vi "LS DAS File Save.vi"(0 "Raw Data":fxp<+/-,22,11>[](array[numeric]), 1 "ValidFifoRead":bool, 2 "Day In":i32, 3 "Count In":i32, 4 "Bank1 Filepath":path, 5 "Bank2 Filepath":path, 6 "Opens In":i32[](array[numeric]), 7 "Row Count In":i32, 8 "Bank2Slow":bool, 9 "LowRate":i32, 10 "Anomaly Filepath":path) -> (15 "Day Out":i32, 18 "Count Out":i32, 19 "Second File Count Out":i32)   [LabVIEW 2013]
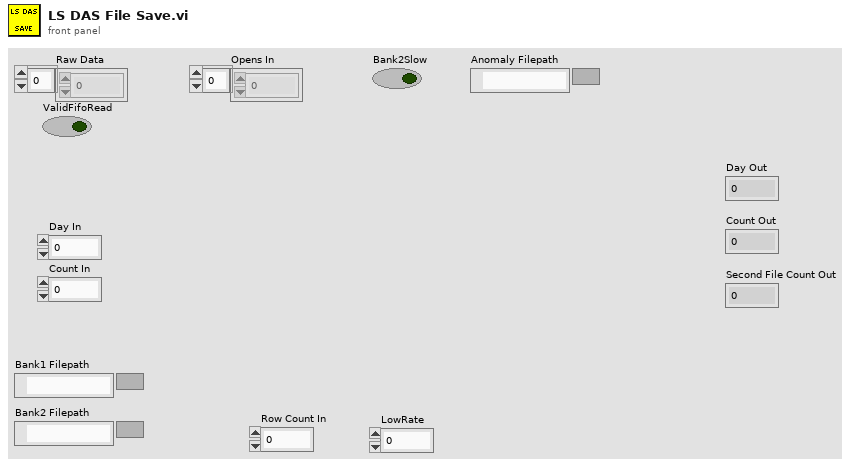
[diagram p1: front panel]
types:
  T1 = enum16{"open", "replace", "create", "open or create", "replace or create", "replace or create with confirmation"}
  T2 = typedef "LVDateTimeRec.ctl" = cluster{"fractional second":dbl, "second":i32, "minute":i32, "hour":i32, "day of month":i32, "month":i32, "year":i32, "day of week":i32, "day of year":i32, "DST":i32}
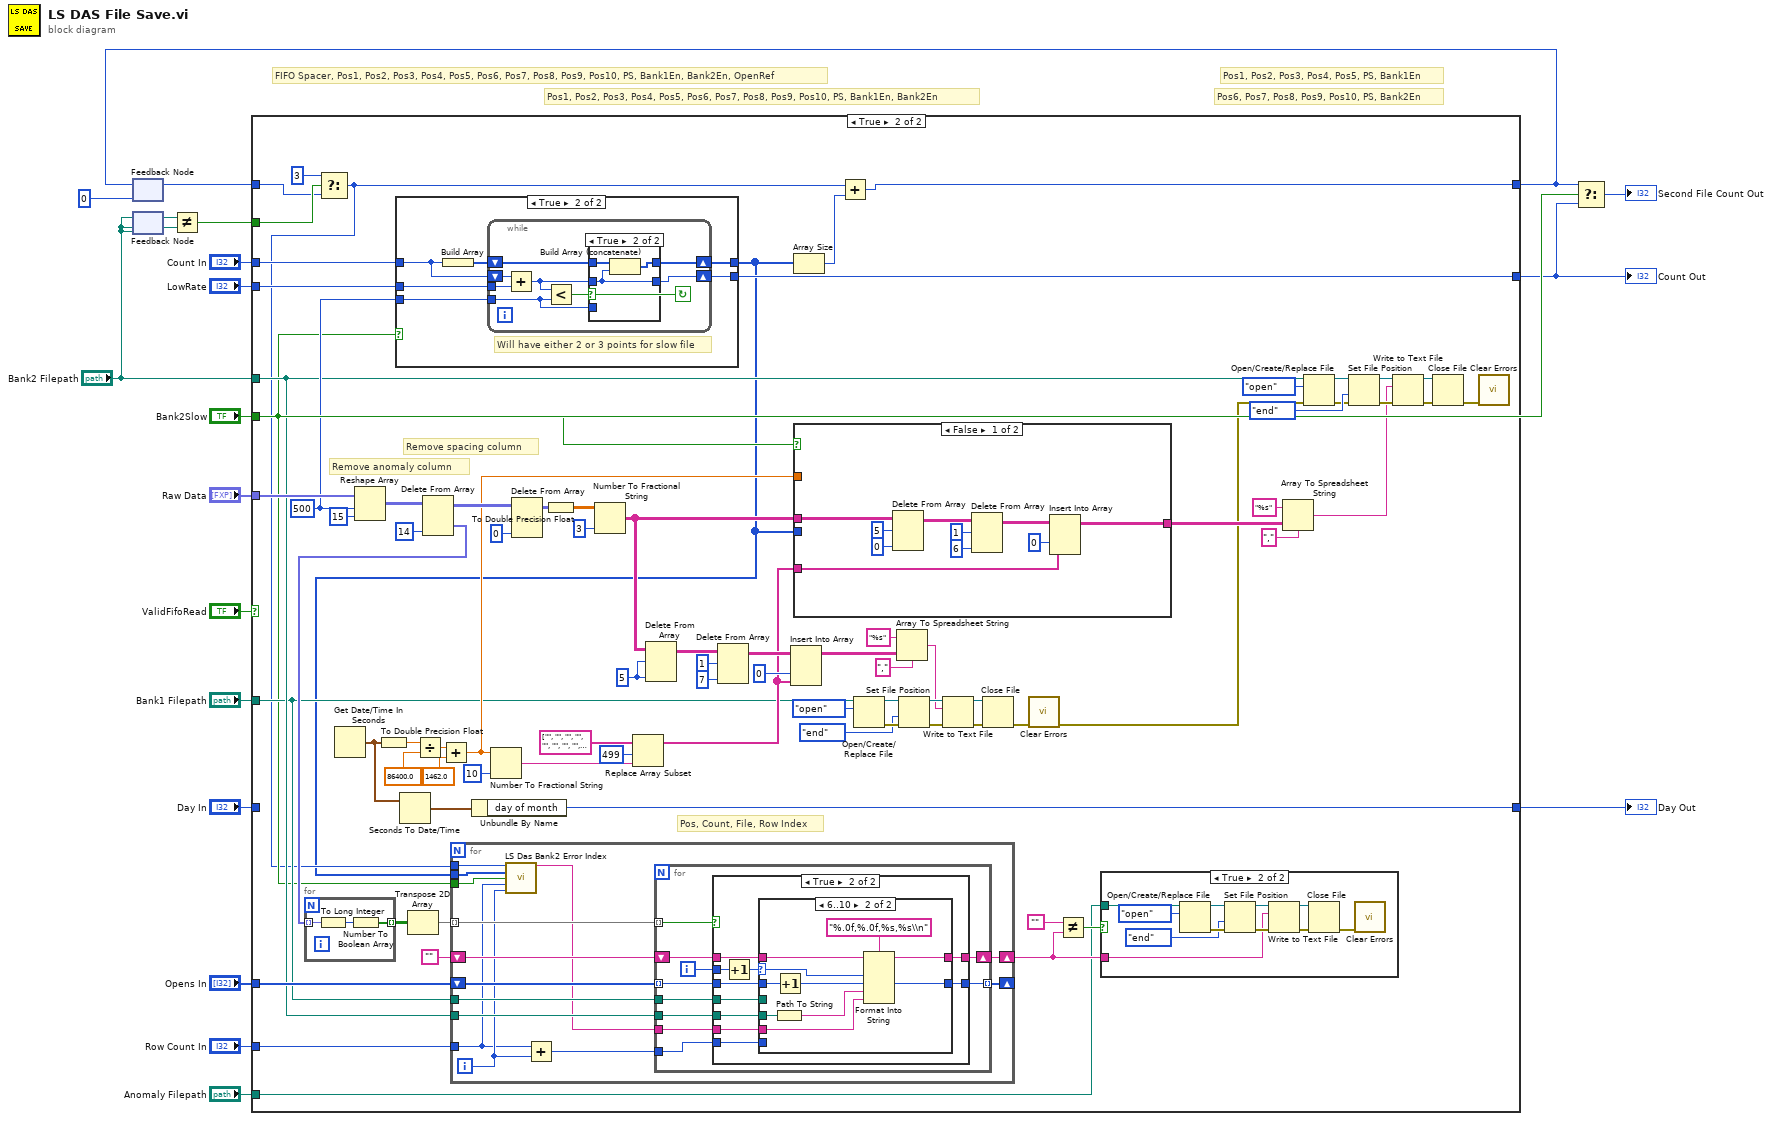
[diagram p0: block diagram]
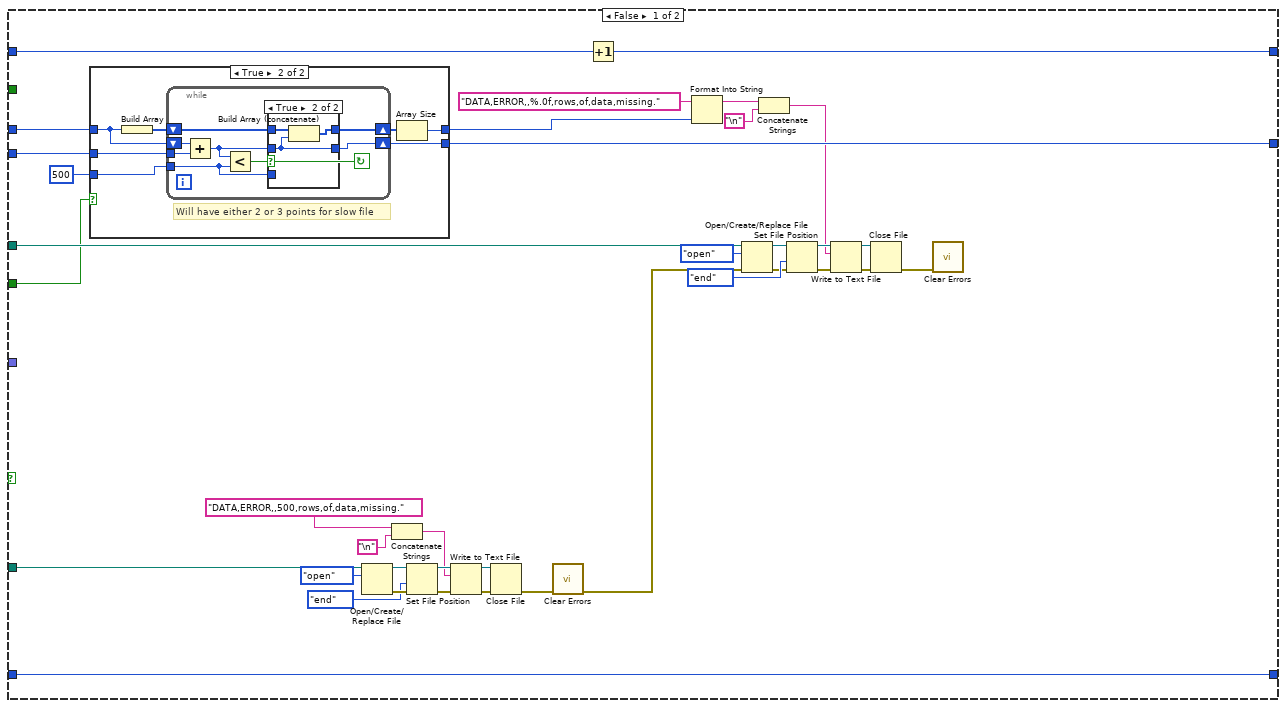
[diagram p2: hidden frame]
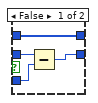
[diagram p4: hidden frame]
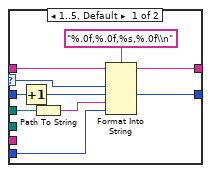
[diagram p7: hidden frame]
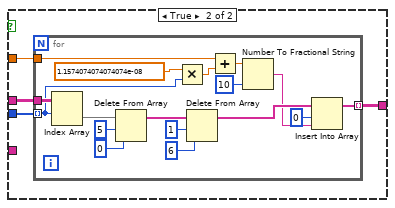
[diagram p8: hidden frame]
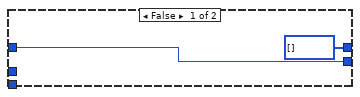
[diagram p9: hidden frame]
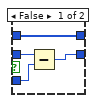
[diagram p10: hidden frame]
diagram:
  # "Pos1, Pos2, Pos3, Pos4, Pos5, Pos6, Pos7, Pos8, Pos9, Pos10, PS, Bank1En, Bank2En"
  # "Pos6, Pos7, Pos8, Pos9, Pos10, PS, Bank2En"
  # "Pos1, Pos2, Pos3, Pos4, Pos5, PS, Bank1En"
  # "FIFO Spacer, Pos1, Pos2, Pos3, Pos4, Pos5, Pos6, Pos7, Pos8, Pos9, Pos10, PS, Bank1En, Bank2En, OpenRef"
  n1 = feedback #1(0) -> (w6:i32)
  n2 = feedback-in #2("Bank2 Filepath") -> ()
  n3 = feedback #2("Bank2 Filepath") -> (w9:path)
  n4 = Not Equal?(x=w9, y="Bank2 Filepath") -> (x != y?=w8:bool)
  n5 = case shown="True" "ValidFifoRead" {
    tunnel: [w52 w156] -> w19
    tunnel: "Raw Data" -> [_ w141]
    tunnel: "Day In" -> [w52 _]
    tunnel: "Bank1 Filepath" -> [w40 w94]
    tunnel: "Bank2 Filepath" -> [w30 w95]
    tunnel: "Count In" -> [w55 w126]
    tunnel: "LowRate" -> [w56 w127]
    tunnel: [w53 w124] -> w2
    tunnel: "Bank2Slow" -> [w22 w91]
    tunnel: "Opens In" -> [_ w96]
    tunnel: "Row Count In" -> [_ w97]
    tunnel: w8 -> [_ w90]
    tunnel: w6 -> [w21 w89]
    tunnel: [w20 w86] -> w3
    tunnel: "Anomaly Filepath" -> [_ w81]
    frame False {
      n6 = case shown="True" w22 {
        tunnel: w56 -> [_ w64]
        tunnel: w55 -> [w57 w63]
        tunnel: 500 ("dimension size") -> [w58 w62]
        tunnel: [w57 w61] -> w53
        tunnel: [w58 w59] -> w26
        frame False {
        }
        frame True {
          # "Will have either 2 or 3 points for slow file"
          n7 = Build Array(w63) -> (w65:i32[])
          n8 = while {
            shift-right: [w69] -> w60
            shift-left: w65 -> [w71]
            tunnel: w64 -> [w72]
            shift-right: [w68] -> w61
            shift-left: w63 -> [w73]
            tunnel: w62 -> [w67]
            stop <- w66 continue-if-true
            n9 = Add(x=w73, y=w72) -> (x+y=w70:i32)
            n10 = Less?(x=w70, y=w67) -> (x < y?=w66:bool)
            n11 = case shown="True" w66 {
              tunnel: w71 -> [w77 w80]
              tunnel: w70 -> [w76 w78]
              tunnel: [w77 w79] -> w69
              tunnel: [w74 w78] -> w68
              tunnel: w67 -> [w75 _]
              frame False {
                n12 = Subtract(x=w76, y=w75) -> (x-y=w74:i32)
              }
              frame True {
                n13 = Build Array (concatenate)(w80, w78) -> (w79:i32[])
              }
            }
          }
          n14 = Array Size(array=w60) -> (size(s)=w59:i32)
        }
      }
      n15 = Open/Create/Replace File(file path (use dialog)=w40, operation (0:open)=T1."open") -> (refnum out=w45:refnum<file>, error out=w44:errorcluster)  [unwired: 4 in, 1 out]
      n16 = Concatenate Strings("DATA,ERROR,,500,rows,of,data,missing." ("string"), "\n") -> (w23:string)
      n17 = Set File Position(refnum=w45, from (0:start)=enum16{"start", "end", "current"}."end", error in=w44) -> (refnum out=w42:refnum<file>, error out=w41:errorcluster)  [unwired: 1 in]
      n18 = Write to Text File(file (use dialog)=w42, text=w23, error in=w41) -> (refnum out=w48:refnum<file>, error out=w49:errorcluster)  [unwired: 1 in, 1 out]
      n19 = Close File(refnum=w48, error in=w49) -> (error out=w47:errorcluster)  [unwired: 1 out]
      n20 = call <vilib>:"Clear Errors.vi"("error in (no error)"=w47) -> ("error out"=w29:errorcluster)  [unwired: 6 in]
      n21 = Increment(x=w21) -> (x+1=w20:i32)
      n22 = Format Into String(initial string="DATA,ERROR,,%.0f,rows,of,data,missing." ("input string"), w26) -> (resulting string=w25:string)  [unwired: 2 in, 1 out]
      n23 = Open/Create/Replace File(file path (use dialog)=w30, error in=w29, operation (0:open)=T1."open") -> (refnum out=w35:refnum<file>, error out=w36:errorcluster)  [unwired: 3 in, 1 out]
      n24 = Concatenate Strings(w25, "\n") -> (w24:string)
      n25 = Set File Position(refnum=w35, from (0:start)=enum16{"start", "end", "current"}."end", error in=w36) -> (refnum out=w38:refnum<file>, error out=w39:errorcluster)  [unwired: 1 in]
      n26 = Write to Text File(file (use dialog)=w38, text=w24, error in=w39) -> (refnum out=w32:refnum<file>, error out=w31:errorcluster)  [unwired: 1 in, 1 out]
      n27 = Close File(refnum=w32, error in=w31) -> (error out=w33:errorcluster)  [unwired: 1 out]
      n28 = call <vilib>:"Clear Errors.vi"("error in (no error)"=w33) -> ()  [unwired: 6 in, 1 out]
    }
    frame True {
      w108 = 5 ("disabled index (col)")
      w125 = 500 ("dimension size")
      # "Pos, Count, File, Row Index"
      # "Remove spacing column"
      # "Remove anomaly column"
      n29 = Select(t=3, s=w90, f=w89) -> (s? t:f=w85:i32)
      n30 = Get Date/Time In Seconds() -> (seconds since 1Jan1904=w146:timestamp)
      n31 = Reshape Array(w141, w125, 15 ("dimension size")) -> (w143:fxp<+/-,22,11>[][])
      n32 = To Double Precision Float(number=w146) -> (double precision float=w148:dbl)
      n33 = case shown="True" w91 {
        tunnel: w127 -> [_ w266]
        tunnel: w126 -> [w261 w265]
        tunnel: w125 -> [_ w264]
        tunnel: [w261 w263] -> w124
        tunnel: [i32[] [] w262] -> w84
        frame False {
        }
        frame True {
          # "Will have either 2 or 3 points for slow file"
          n34 = Build Array(w265) -> (w267:i32[])
          n35 = while {
            shift-right: [w271] -> w262
            shift-left: w267 -> [w273]
            tunnel: w266 -> [w274]
            shift-right: [w270] -> w263
            shift-left: w265 -> [w275]
            tunnel: w264 -> [w269]
            stop <- w268 continue-if-true
            n36 = Add(x=w275, y=w274) -> (x+y=w272:i32)
            n37 = Less?(x=w272, y=w269) -> (x < y?=w268:bool)
            n38 = case shown="True" w268 {
              tunnel: w273 -> [w279 w282]
              tunnel: w272 -> [w278 w280]
              tunnel: [w279 w281] -> w271
              tunnel: [w276 w280] -> w270
              tunnel: w269 -> [w277 _]
              frame False {
                n39 = Subtract(x=w278, y=w277) -> (x-y=w276:i32)
              }
              frame True {
                n40 = Build Array (concatenate)(w282, w280) -> (w281:i32[])
              }
            }
          }
        }
      }
      n41 = Seconds To Date/Time(time stamp (now)=w146) -> (date time rec=w145:T2)  [unwired: 1 in]
      n42 = Divide(x=w148, y=86400.0) -> (x/y=w150:dbl)
      n43 = Delete From Array(array=w143, index (col)=14 ("disabled index (col)")) -> (deleted portion=w100:fxp<+/-,22,11>[], array with subset deleted=w157:fxp<+/-,22,11>[][])  [unwired: 2 in]
      n44 = for {
        tunnel: w100 -> [w228] mode=indexing
        tunnel: [w226] -> w99 mode=indexing
        n45 = To Long Integer(number=w228) -> (32bit integer=w227:i32)
        n46 = Number To Boolean Array(number=w227) -> (Boolean array=w226:bool[])
      }
      n47 = Transpose 2D Array(2D array=w99) -> (transposed array=w98:bool[][])
      n48 = Add(x=w150, y=1462.0) -> (x+y=w110:dbl)
      n49 = for {
        tunnel: w98 -> [w185] mode=indexing
        tunnel: w97 -> [w173]
        shift-right: [w184] -> _
        shift-left: w96 -> [w183]
        tunnel: w95 -> [w182]
        tunnel: w94 -> [w181]
        shift-right: [w179] -> w82
        shift-left: "" -> [w180]
        tunnel: w91 -> [w172]
        tunnel: w85 -> [w177]
        tunnel: w84 -> [w176]
        i -> [w174]
        n50 = call "LS Das Bank2 Error Index.vi"("RowCountSlow"=w177, "SlowRecordIndexes"=w176, "Bank2SlowRecord"=w172, "RowCountStandard"=w173, "ErrorIndex"=w174) -> ("Bank2ErrorIndex"=w175:string)  [unwired: 10 in]
        n51 = Add(x=w173, y=w174) -> (x+y=w178:i32)
        n52 = for {
          tunnel: w185 -> [w194] mode=indexing
          tunnel: w183 -> [w193] mode=indexing
          tunnel: [w192] -> w184 mode=indexing
          tunnel: w182 -> [w191]
          tunnel: w181 -> [w190]
          shift-right: [w188] -> w179
          shift-left: w180 -> [w189]
          tunnel: w178 -> [w187]
          tunnel: w175 -> [w186]
          i -> [w195]
          n53 = case shown="True" w194 {
            tunnel: w195 -> [_ w201]
            tunnel: w193 -> [w196 w207]
            tunnel: [w196 w206] -> w192
            tunnel: w191 -> [_ w205]
            tunnel: w190 -> [_ w204]
            tunnel: w189 -> [w197 w203]
            tunnel: [w197 w202] -> w188
            tunnel: w187 -> [_ w199]
            tunnel: w186 -> [_ w198]
            frame False {
            }
            frame True {
              n54 = Increment(x=w201) -> (x+1=w200:i32)
              n55 = case shown="6..10" w200 {
                selector: w200 -> [w211 w220]
                tunnel: w207 -> [w215 w224]
                tunnel: [w214 w223] -> w206
                tunnel: w205 -> [_ w218]
                tunnel: w204 -> [w208 _]
                tunnel: w203 -> [w213 w222]
                tunnel: [w212 w221] -> w202
                tunnel: w199 -> [w209 _]
                tunnel: w198 -> [_ w217]
                frame 1..5, Default {
                  n56 = Increment(x=w215) -> (x+1=w214:i32)
                  n57 = Path To String(path=w208) -> (string=w210:string)
                  n58 = Format Into String(format string="%.0f,%.0f,%s,%.0f\\n" ("initial string"), initial string=w213, w211, w214, w210, w209) -> (resulting string=w212:string)  [unwired: 1 in, 1 out]
                }
                frame 6..10 {
                  n59 = Path To String(path=w218) -> (string=w219:string)
                  n60 = Increment(x=w224) -> (x+1=w223:i32)
                  n61 = Format Into String(format string="%.0f,%.0f,%s,%s\\n" ("initial string"), initial string=w222, w220, w223, w219, w217) -> (resulting string=w221:string)  [unwired: 1 in, 1 out]
                }
              }
            }
          }
        }
      }
      n62 = Unbundle By Name(w145) -> ("day of month"=w156:i32)
      n63 = Number To Fractional String(number=w110, precision (6)=i16 10) -> (F-format string=w147:string)  [unwired: 2 in]
      n64 = Delete From Array(array=w157, index (col)=0 ("disabled index (col)")) -> (array with subset deleted=w159:fxp<+/-,22,11>[][])  [unwired: 2 in, 1 out]
      n65 = To Double Precision Float(number=w159) -> (double precision float=w160:dbl[][])
      n66 = Number To Fractional String(number=w160, precision (6)=i16 3) -> (F-format string=w103:string[][])  [unwired: 2 in]
      n67 = Replace Array Subset(array=string[] ["", "", "", "", "", "", "", "", "", "", "", "", "", "", "", "", "", "", "", "", "", "", "", "", "", "", "", "", "", "", "", "", "", "", "", "", "", "", "", "", "", "", "", "", "", "", "", "", "", "", "", "", "", "", "", "", "", "", "", "", "", "", "", "", "", "", "", "", "", "", "", "", "", "", "", "", "", "", "", "", "", "", "", "", "", "", "", "", "", "", "", "", "", "", "", "", "", "", "", "", "", "", "", "", "", "", "", "", "", "", "", "", "", "", "", "", "", "", "", "", "", "", "", "", "", "", "", "", "", "", "", "", "", "", "", "", "", "", "", "", "", "", "", "", "", "", "", "", "", "", "", "", "", "", "", "", "", "", "", "", "", "", "", "", "", "", "", "", "", "", "", "", "", "", "", "", "", "", "", "", "", "", "", "", "", "", "", "", "", "", "", "", "", "", "", "", "", "", "", "", "", "", "", "", "", "", "", "", "", "", "", "", "", "", "", "", "", "", "", "", "", "", "", "", "", "", "", "", "", "", "", "", "", "", "", "", "", "", "", "", "", "", "", "", "", "", "", "", "", "", "", "", "", "", "", "", "", "", "", "", "", "", "", "", "", "", "", "", "", "", "", "", "", "", "", "", "", "", "", "", "", "", "", "", "", "", "", "", "", "", "", "", "", "", "", "", "", "", "", "", "", "", "", "", "", "", "", "", "", "", "", "", "", "", "", "", "", "", "", "", "", "", "", "", "", "", "", "", "", "", "", "", "", "", "", "", "", "", "", "", "", "", "", "", "", "", "", "", "", "", "", "", "", "", "", "", "", "", "", "", "", "", "", "", "", "", "", "", "", "", "", "", "", "", "", "", "", "", "", "", "", "", "", "", "", "", "", "", "", "", "", "", "", "", "", "", "", "", "", "", "", "", "", "", "", "", "", "", "", "", "", "", "", "", "", "", "", "", "", "", "", "", "", "", "", "", "", "", "", "", "", "", "", "", "", "", "", "", "", "", "", "", "", "", "", "", "", "", "", "", "", "", "", "", "", "", "", "", "", "", "", "", "", "", "", "", "", "", "", "", "", "", "", "", "", "", "", "", "", "", "", "", "", "", "", "", "", "", "", "", "", "", "", "", "", "", "", "", "", ""], new element=w147, index=499) -> (w101:string[])
      n68 = Delete From Array(array=w103, length=w108, index (col)=w108) -> (array with subset deleted=w107:string[][])  [unwired: 1 in, 1 out]
      n69 = Delete From Array(array=w107, length=1, index (col)=7 ("disabled index (col)")) -> (array with subset deleted=w104:string[][])  [unwired: 1 in, 1 out]
      n70 = Insert Into Array(array=w104, index (col)=0 ("disabled index (col)"), new element=w101) -> (w102:string[][])  [unwired: 1 in]
      n71 = Array Size(array=w84) -> (size(s)=w87:i32)
      n72 = case shown="False" w91 {
        tunnel: w103 -> [w238 w242]
        tunnel: [w232 w241] -> w112
        tunnel: w110 -> [_ w240]
        tunnel: w84 -> [_ w239]
        tunnel: w101 -> [w230 _]
        frame False {
          n73 = Delete From Array(array=w238, length=5, index (col)=0 ("disabled index (col)")) -> (array with subset deleted=w235:string[][])  [unwired: 1 in, 1 out]
          n74 = Delete From Array(array=w235, length=1, index (col)=6 ("disabled index (col)")) -> (array with subset deleted=w233:string[][])  [unwired: 1 in, 1 out]
          n75 = Insert Into Array(array=w233, index (col)=0 ("disabled index (col)"), new element=w230) -> (w232:string[][])  [unwired: 1 in]
        }
        frame True {
          n76 = for {
            tunnel: w239 -> [w255] mode=indexing
            tunnel: w242 -> [w259]
            tunnel: w240 -> [w256]
            tunnel: [w245] -> w241 mode=indexing
            n77 = Index Array(array=w259, index (row)=w255) -> (element=w249:string[])  [unwired: 1 in]
            n78 = Delete From Array(array=w249, length=5, index=0) -> (array with subset deleted=w248:string[])  [unwired: 1 out]
            n79 = Multiply(x=1.1574074074074074e-08, y=w255) -> (x*y=w254:dbl)
            n80 = Delete From Array(array=w248, length=1 ("index"), index=6 ("length")) -> (array with subset deleted=w247:string[])  [unwired: 1 out]
            n81 = Add(x=w256, y=w254) -> (x+y=w253:dbl)
            n82 = Number To Fractional String(number=w253, precision (6)=i16 10) -> (F-format string=w246:string)  [unwired: 2 in]
            n83 = Insert Into Array(array=w247, index=0, new element=w246) -> (w245:string[])
          }
        }
      }
      n84 = Add(x=w85, y=w87) -> (x+y=w86:i32)
      n85 = Open/Create/Replace File(file path (use dialog)=w94, operation (0:open)=T1."open") -> (refnum out=w135:refnum<file>, error out=w134:errorcluster)  [unwired: 4 in, 1 out]
      n86 = Array To Spreadsheet String(delimiter (Tab)=",", array=w102, 3:"%s" ("format string")) -> (spreadsheet string=w128:string)
      n87 = Set File Position(refnum=w135, from (0:start)=enum16{"start", "end", "current"}."end", error in=w134) -> (refnum out=w132:refnum<file>, error out=w131:errorcluster)  [unwired: 1 in]
      n88 = Write to Text File(file (use dialog)=w132, text=w128, error in=w131) -> (refnum out=w138:refnum<file>, error out=w139:errorcluster)  [unwired: 1 in, 1 out]
      n89 = Close File(refnum=w138, error in=w139) -> (error out=w137:errorcluster)  [unwired: 1 out]
      n90 = call <vilib>:"Clear Errors.vi"("error in (no error)"=w137) -> ("error out"=w109:errorcluster)  [unwired: 6 in]
      n91 = Not Equal?(x="", y=w82) -> (x != y?=w83:bool)
      n92 = case shown="True" w83 {
        tunnel: w82 -> [_ w162]
        tunnel: w81 -> [_ w161]
        frame False {
        }
        frame True {
          n93 = Open/Create/Replace File(file path (use dialog)=w161, operation (0:open)=T1."open") -> (refnum out=w167:refnum<file>, error out=w166:errorcluster)  [unwired: 4 in, 1 out]
          n94 = Set File Position(refnum=w167, from (0:start)=enum16{"start", "end", "current"}."end", error in=w166) -> (refnum out=w164:refnum<file>, error out=w163:errorcluster)  [unwired: 1 in]
          n95 = Write to Text File(file (use dialog)=w164, text=w162, error in=w163) -> (refnum out=w170:refnum<file>, error out=w171:errorcluster)  [unwired: 1 in, 1 out]
          n96 = Close File(refnum=w170, error in=w171) -> (error out=w169:errorcluster)  [unwired: 1 out]
          n97 = call <vilib>:"Clear Errors.vi"("error in (no error)"=w169) -> ()  [unwired: 6 in, 1 out]
        }
      }
      n98 = Array To Spreadsheet String(delimiter (Tab)=",", array=w112, 3:"%s" ("format string")) -> (spreadsheet string=w111:string)
      n99 = Open/Create/Replace File(file path (use dialog)=w95, error in=w109, operation (0:open)=T1."open") -> (refnum out=w119:refnum<file>, error out=w120:errorcluster)  [unwired: 3 in, 1 out]
      n100 = Set File Position(refnum=w119, from (0:start)=enum16{"start", "end", "current"}."end", error in=w120) -> (refnum out=w122:refnum<file>, error out=w123:errorcluster)  [unwired: 1 in]
      n101 = Write to Text File(file (use dialog)=w122, text=w111, error in=w123) -> (refnum out=w116:refnum<file>, error out=w115:errorcluster)  [unwired: 1 in, 1 out]
      n102 = Close File(refnum=w116, error in=w115) -> (error out=w117:errorcluster)  [unwired: 1 out]
      n103 = call <vilib>:"Clear Errors.vi"("error in (no error)"=w117) -> ()  [unwired: 6 in, 1 out]
    }
  }
  "Day Out" <- w19
  "Count Out" <- w2
  n104 = feedback-in #1(w3) -> ()
  n105 = Select(t=w3, s="Bank2Slow", f=w2) -> (s? t:f=→"Second File Count Out":i32)
